vi "Print Session Scope.vi"(8 "error in (no error)":errorcluster, 11 "Session Handle in":refnum<data-value>) -> (0 "error out":errorcluster, 1 "String":string, 3 "Session Handle out":refnum<data-value>)   [LabVIEW 2020, in "G-Embedded-Python-Interpreter-Toolkit.lvlib"]
uses:
  G-Embedded-Python-Interpreter-Toolkit.lvlib
  bin/gepit.cp310.32.dll
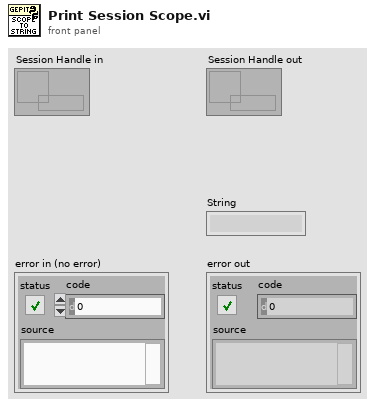
[diagram p1: front panel]
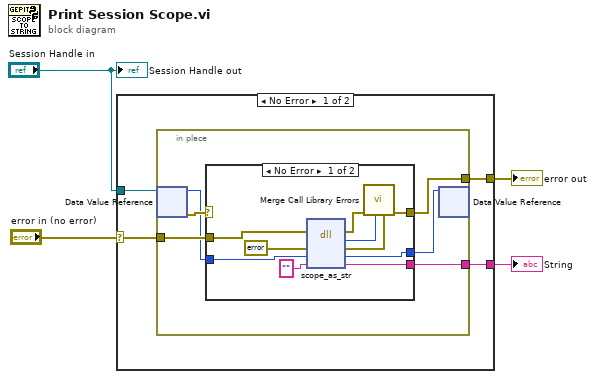
[diagram p0: block diagram]
diagram:
  n1 = case shown="No Error" "error in (no error)" {
    selector: "error in (no error)" -> [w7 w27]
    tunnel: "Session Handle in" -> [w8 _]
    tunnel: [w6 w27] -> w3
    tunnel: [w5 _] -> w1
    frame No Error {
      n2 = in-place {
        in-place-border: w7 -> [w13]
        in-place-border: [w10] -> w6
        in-place-border: [w9] -> w5
        n3 = in-place-dvr #1(w8) -> (w12:u64, w14:errorcluster)
        n4 = case shown="No Error" w14 {
          selector: w14 -> [_ w25]
          tunnel: w13 -> [w20 _]
          tunnel: w12 -> [w19 w26]
          tunnel: [w18 w26] -> w11
          tunnel: [w17 w25] -> w10
          tunnel: [w15 _] -> w9
          frame No Error {
            n5 = dll-call lib="C:/serenial/libraries/g-embedded-python-interpreter-toolkit/LabVIEW/bin/gepit.cp310.32.dll" fn="scope_as_str"(error in=w20, "Error"=errorcluster {"status"=FALSE, "code"=0, "source"=""} ("error constant"), "Session"=w19, "String"="") -> (error out=w23:errorcluster, "return type"=w22:i32, "Error"=w21:errorcluster, "Session"=w18:u64, "String"=w15:string)  [unwired: 2 in, 1 out]
            n6 = call "Merge Call Library Errors.vi"("Call Library Error"=w21, "Return Value"=w22, "error in"=w23) -> ("error out"=w17:errorcluster)  [unwired: 8 in]
          }
          frame Error {
          }
        }
        n7 = in-place-dvr #1(w11) -> ()  [unwired: 2 out]
      }
    }
    frame Error {
    }
  }
  "error out" <- w3
  "String" <- w1
  "Session Handle out" <- "Session Handle in"
